vi "Dynamic Dispatching.vi"() -> ()   [LabVIEW 2023]
doc: "Demonstrates dynamic dispatching with LabVIEW classes."
uses:
  Square/Square.lvclass
  c:/dev/_r/4/eng/lv-core/lvpostprocessingd/lv_mc_x86_64/dist_i386/examples/Object-Oriented Programming/Dynamic Dispatching/Shape/Shape.lvclass
  Shape/Shape.lvclass
  Triangle/Triangle.lvclass
panel:
  out "names":string[](array[string])
  # "Overview: Demonstrates dynamic dispatching with LabVIEW classes.\nInstructions:\n1. Run the VI to see the list of LabVIEW class names.\n2. Open the block diagram and refer to the comments there."
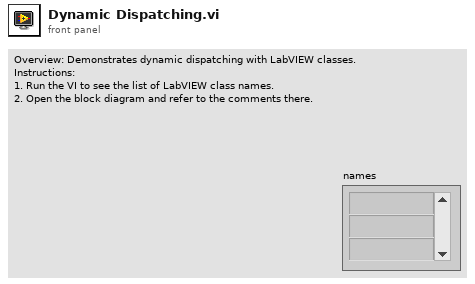
[diagram p1: front panel]
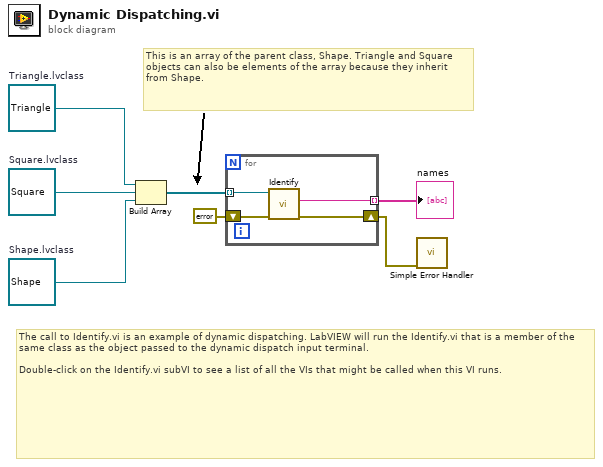
[diagram p0: block diagram]
diagram:
  w1 = refnum<class "Triangle.lvclass"> refnum  # Triangle.lvclass
  w4 = refnum<class "Shape.lvclass"> refnum  # Shape.lvclass
  w5 = refnum<class "Square.lvclass"> refnum  # Square.lvclass
  # "This is an array of the parent class, Shape. Triangle and Square objects can also be elements of the array because they inherit from Shape."
  # "The call to Identify.vi is an example of dynamic dispatching. LabVIEW will run the Identify.vi that is a member of the same class as the object passed to the dynamic dispatch input terminal.\n\nDouble-click on the Identify.vi subVI to see a list of all the VIs that might be called when this VI runs."
  n1 = Build Array(w1, w5, w4) -> (w7:refnum<class "Shape.lvclass">[])
  n2 = for {
    tunnel: w7 -> [w11] mode=indexing
    tunnel: [w10] -> w6 mode=indexing
    shift-right: [w9] -> w3
    shift-left: errorcluster {"status"=FALSE, "code"=0, "source"=""} ("error out") -> [w8]
    n3 = call-dynamic "Identify.vi"("error in (no error)"=w8, "Shape in"=w11) -> ("error out"=w9:errorcluster, "Class name"=w10:string)  [unwired: 7 in, 1 out]
  }
  "names" <- w6
  n4 = call <vilib>:"Simple Error Handler.vi"("error in (no error)"=w3) -> ()  [unwired: 4 in, 5 out]
